vi "FTP_Start.vi"(0 "address":string, 1 "remote port (21)":u16=21, 3 "error in (no error)":errorcluster, 4 "local port":u16) -> (5 "connection ID":refnum<k5>, 6 "Good Reply?":bool, 7 "error out":errorcluster)   [LabVIEW 2012]
uses:
  <userlib>/BotSpeak/Devices/EvalRIO/FTPCodes/FTPGlobals.vi
panel:
  out "reply string":string
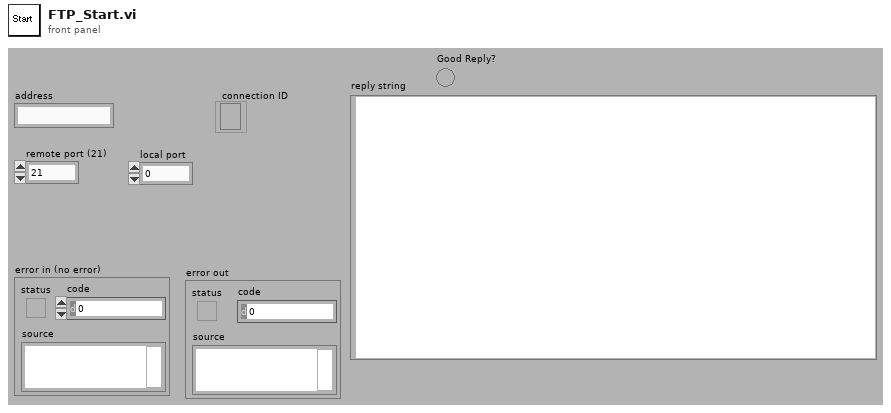
[diagram p1: front panel]
types:
  T1 = enum16{"unknown", "100 + Prelim", "200 + ", "300 + Intermed", "400 - Transient", "500 - Permanent"}
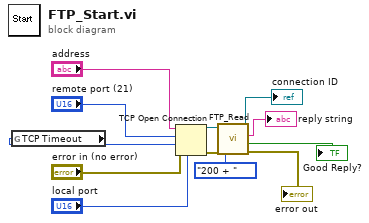
[diagram p0: block diagram]
diagram:
  n1 = global read "FTPGlobals.vi" "TCP Timeout"() -> (w1:i32)
  n2 = TCP Open Connection(address="address", remote port or service name="remote port (21)", timeout ms (60000)=w1, local port="local port", error in (no error)="error in (no error)") -> (connection ID=w4:refnum<k5>, error out=w6:errorcluster)
  n3 = call <userlib>:"FTP_Read.vi"("error In"=w6, "expected class"=T1."200 + ", "connection ID"=w4) -> ("error out"=→"error out":errorcluster, "Good Reply?"=→"Good Reply?":bool, "reply string"=→"reply string":string, "connection ID out"=→"connection ID":refnum<k5>)  [unwired: 1 out]
